vi "set_ellipse.vi"(0 "Set/Add":bool, 1 "y2":dbl, 2 "y1":dbl, 3 "Handle":i32, 4 "x2":dbl, 5 "x1":dbl) -> ()   [LabVIEW 2010]
uses:
  MWT_1.3.0_r1035/MultiWorm Tracker v1.3.0/data/MWT.dll
panel:
  out "radius y":dbl
  out "radius x":dbl
  out "center y":dbl
  out "center x":dbl
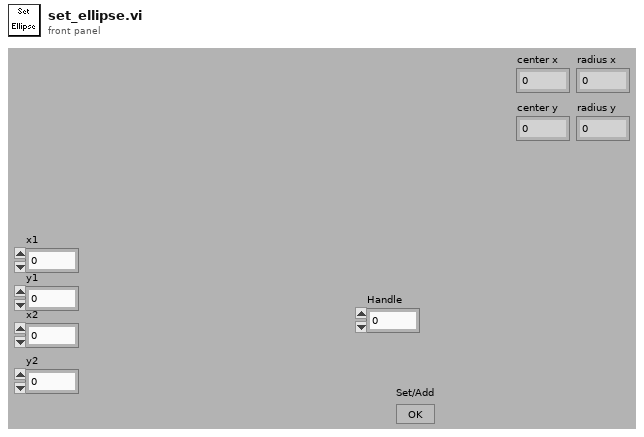
[diagram p1: front panel]
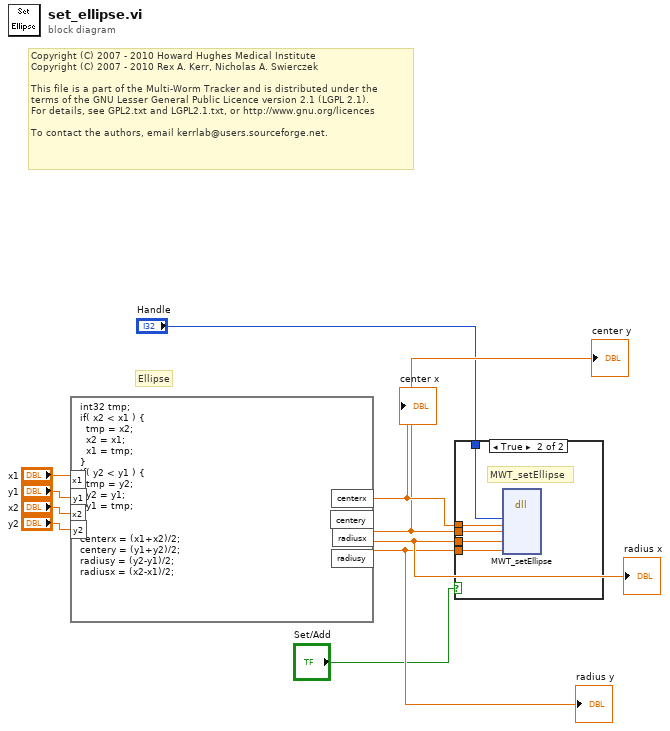
[diagram p0: block diagram]
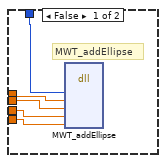
[diagram p2: hidden frame]
diagram:
  # "Copyright (C) 2007 - 2010 Howard Hughes Medical Institute\nCopyright (C) 2007 - 2010 Rex A. Kerr, Nicholas A. Swierczek\n \nThis file is a part of the Multi-Worm Tracker and is distributed under the\nterms of the GNU Lesser General Public Licence version 2.1 (LGPL 2.1).\nFor details, see GPL2.txt and LGPL2.1.txt, or http://www.gnu.org/licences\n \nTo contact the authors, email kerrlab@users.sourceforge.net."
  # "Ellipse"
  n1 = formula code="int32 tmp;\nif( x2 < x1 ) {\n  tmp = x2;\n  x2 = x1;\n  x1 = tmp;\n}\nif( y2 < y1 ) {\n  tmp = y2;\n  y2 = y1;\n  y1 = tmp;\n}\n\ncenterx = (x1+x2)/2;\ncentery = (y1+y2)/2;\nradiusy = (y2-y1)/2;\nradiusx = (x2-x1)/2;"("x1"="x1", "y1"="y1", "x2"="x2", "y2"="y2") -> ("centerx"=w10:dbl, "centery"=w9:dbl, "radiusx"=w8:dbl, "radiusy"=w7:dbl)
  "center x" <- w10
  "center y" <- w9
  "radius x" <- w8
  "radius y" <- w7
  n2 = case shown="True" "Set/Add" {
    tunnel: w10 -> [w15 w20]
    tunnel: w9 -> [w14 w19]
    tunnel: w8 -> [w13 w18]
    tunnel: w7 -> [w12 w17]
    tunnel: "Handle" -> [w11 w16]
    frame False {
      # "MWT_addEllipse"
      n3 = dll-call lib="C:/Users/Marc/multi worm tracker/MWT_1.3.0_r1035/MultiWorm Tracker v1.3.0/data/MWT.dll" fn="MWT_addEllipse"("handle"=w11, "centerx"=w15, "centery"=w14, "radiusx"=w13, "radiusy"=w12) -> ()  [unwired: 9 in, 2 out]
    }
    frame True {
      # "MWT_setEllipse"
      n4 = dll-call lib="C:/Users/Marc/multi worm tracker/MWT_1.3.0_r1035/MultiWorm Tracker v1.3.0/data/MWT.dll" fn="MWT_setEllipse"("handle"=w16, "centerx"=w20, "centery"=w19, "radiusx"=w18, "radiusy"=w17) -> ()  [unwired: 9 in, 2 out]
    }
  }
